vi "Create Notification Icon.vi"(11 "error in (no error)":errorcluster) -> (4 "NotifyIcon out":refnum<class "NotifyIcon.lvclass">, 10 "Notify Icon Event":refnum<user-event>, 15 "error out":errorcluster)   [LabVIEW 2018, in "NotifyIcon.lvclass"]
doc: "This VI creates a new NotifyIcon Class instance.\nUse the <b>Notify Icon Event</b> output to dynamically register user events generated when a user interact with the Notification Icon and the associated Context Menu.\n\n\nStinus Olsen\nCIM Industrial Systems A/S\n22. Feb. 2011 15:04\nmailto: seo@cim.as"
uses:
  NotifyIcon.lvclass
  Controls/Notify Event.ctl
  Controls/Notify Event Type.ctl
  System.Windows.Forms
  NotifyIcon.lvclass/NotifyIcon.ctl
panel:
  # "This VI belongs to the NotifyIcon Toolset. \nA toolset that makes it easy to create, control and manipulate a notification icon in the notification area of the Windows taskbar.\nThe toolset requires Microsoft .NET framework 2.0\n\n\nNOTICE -- YOU MUST LEAVE THIS NOTICE IN PLACE.  PER THE TERMS OF THE LICENSE BELOW, YOU MAY SUBLICENSE THIS SOFTWARE \nIN ANY WAY THAT DOES NOT CONFLICT WITH THIS LICENSE.\n\n### BSD License (http://www.opensource.org/licenses/bsd-license.php) Begin ###\n \nCopyright (c) 2011, Stinus Olsen <seo@cim.as>\n\nAll rights reserved.\n\nRedistribution and use in source and binary forms, with or without modification, are permitted provided that the following conditions are met:\n\n    * Redistributions of source code must retain the above copyright notice, this list of conditions and the following disclaimer.\n    * Redistributions in binary form must reproduce the above copyright notice, this list of conditions and the following disclaimer in the \n       documentation and/or other materials provided with the distribution.\n    * Neither the name of CIM Industrial Systems nor the names of its contributors may be used to endorse or promote products derived \n       from this software without specific prior written permission.\n\nTHIS SOFTWARE IS PROVIDED BY THE COPYRIGHT HOLDERS AND CONTRIBUTORS \"AS IS\" AND ANY EXPRESS OR IMPLIED WARRANTIES, \nINCLUDING, BUT NOT LIMITED TO, THE IMPLIED WARRANTIES OF MERCHANTABILITY AND FITNESS FOR A PARTICULAR PURPOSE ARE \nDISCLAIMED. IN NO EVENT SHALL THE COPYRIGHT OWNER OR CONTRIBUTORS BE LIABLE FOR ANY DIRECT, INDIRECT, INCIDENTAL,\n SPECIAL, EXEMPLARY, OR CONSEQUENTIAL DAMAGES (INCLUDING, BUT NOT LIMITED TO, PROCUREMENT OF SUBSTITUTE GOODS OR \nSERVICES; LOSS OF USE, DATA, OR PROFITS; OR BUSINESS INTERRUPTION) HOWEVER CAUSED AND ON ANY THEORY OF LIABILITY, \nWHETHER IN CONTRACT, STRICT LIABILITY, OR TORT (INCLUDING NEGLIGENCE OR OTHERWISE) ARISING IN ANY WAY OUT OF THE USE \nOF THIS SOFTWARE, EVEN IF ADVISED OF THE POSSIBILITY OF SUCH DAMAGE.\n\n### BSD License End ###"
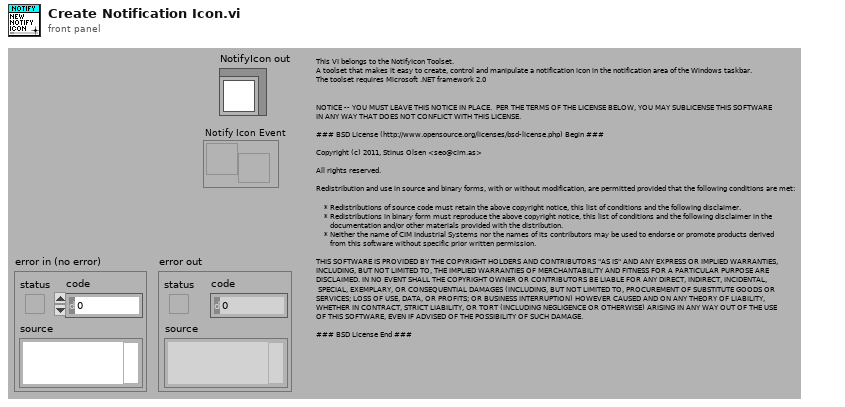
[diagram p1: front panel]
types:
  T1 = typedef "NotifyIcon.lvclass/Notify Event.ctl" = cluster{"Type":T2, "Tag":string}
  T2 = typedef "NotifyIcon.lvclass/Notify Event Type.ctl" = enum16{"<Invalid Event>", "Tray Icon Click", "Tray Icon DoubleClick", "BalloonTip Shown", "BalloonTip Clicked", "BalloonTip Closed", "Menu Item Clicked"}
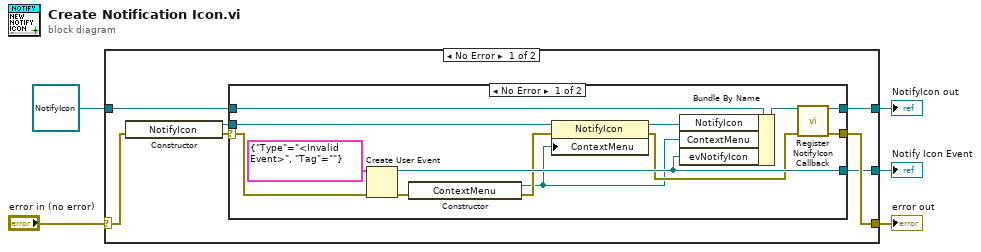
[diagram p0: block diagram]
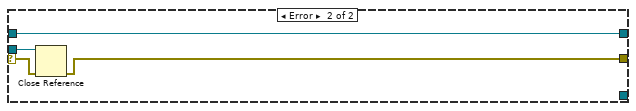
[diagram p2: hidden frame]
diagram:
  n1 = case shown="No Error" "error in (no error)" {
    selector: "error in (no error)" -> [w12 w31]
    tunnel: [w7 w31] -> w4
    tunnel: [w9 w30] -> w3
    tunnel: refnum<class "NotifyIcon.lvclass"> refnum ("Notify Icon.lvclass") -> [w10 w30]
    tunnel: [w6 _] -> w1
    frame No Error {
      n2 = constructor class="NotifyIcon"(error in=w12) -> (reference out=w11:refnum<k24>, error out=w8:errorcluster)  [unwired: 2 in, 1 out]
      n3 = case shown="No Error" w8 {
        selector: w8 -> [w24 w27]
        tunnel: w11 -> [w19 w28]
        tunnel: w10 -> [w25 w29]
        tunnel: [w14 w29] -> w9
        tunnel: [w13 w26] -> w7
        tunnel: [w20 _] -> w6
        frame No Error {
          n4 = Create User Event(user event datatype=T1 {"Type"=enum."<Invalid Event>", "Tag"=""} ("Notify Icon Event"), error in=w24) -> (user event=w20:refnum<user-event>, error out=w21:errorcluster)
          n5 = constructor class="ContextMenu"(error in=w21) -> (reference out=w15:refnum<k24>, error out=w17:errorcluster)  [unwired: 2 in, 1 out]
          n6 = property class="NotifyIcon"(reference=w19, error in=w17, "ContextMenu"=w15) -> (reference out=w18:refnum<k24>, error out=w16:errorcluster)
          n7 = Bundle By Name(cluster=w25, "NotifyIcon"=w18, "ContextMenu"=w15, "evNotifyIcon"=w20) -> (w22:refnum<class "NotifyIcon.lvclass">)
          n8 = call "Register NotifyIcon Callback.vi"("NotifyIcon in"=w22, "error in (no error)"=w16) -> ("NotifyIcon out"=w14:refnum<class "NotifyIcon.lvclass">, "error out"=w13:errorcluster)  [unwired: 12 out]
        }
        frame Error {
          n9 = Close Reference(reference=w28, error in (no error)=w27) -> (error out=w26:errorcluster)
        }
      }
    }
    frame Error {
    }
  }
  "error out" <- w4
  "NotifyIcon out" <- w3
  "Notify Icon Event" <- w1
